vi "subplot_type.vi"(10 "数组":refnum<vi>[](array[refnum]), 11 "枚举":enum16{"1", "11", "1/1", "12", "1/2", "2/2"}(ring)) -> ()   [LabVIEW 2018, in "UI.lvlib"]
uses:
  UI.lvlib
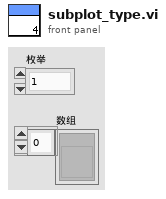
[diagram p1: front panel]
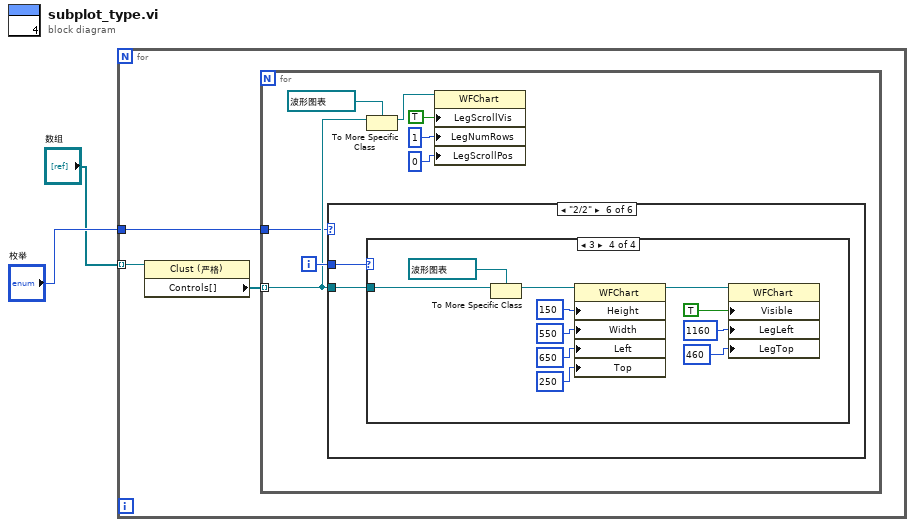
[diagram p0: block diagram]
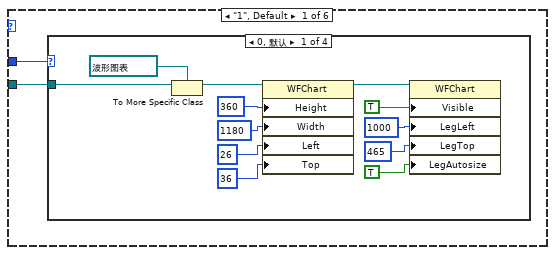
[diagram p2: hidden frame]
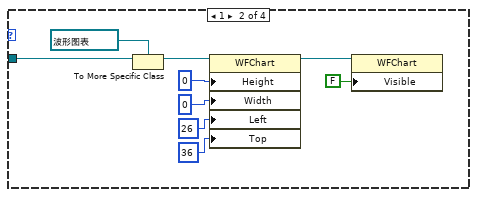
[diagram p3: hidden frame]
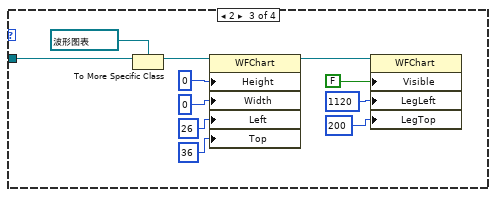
[diagram p4: hidden frame]
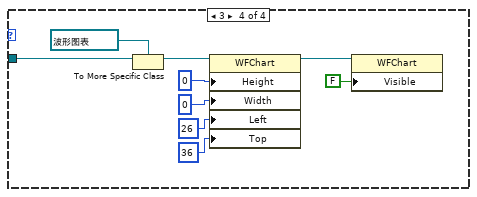
[diagram p5: hidden frame]
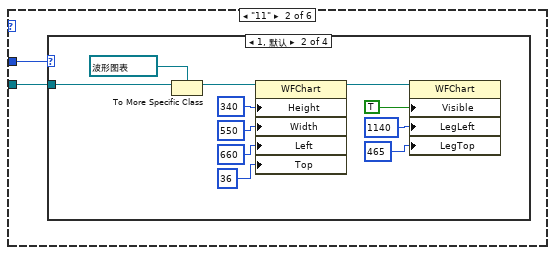
[diagram p6: hidden frame]
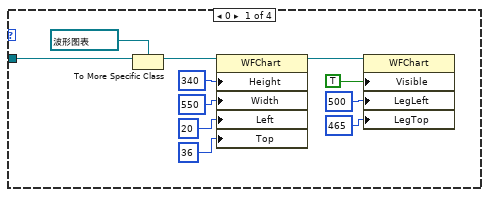
[diagram p7: hidden frame]
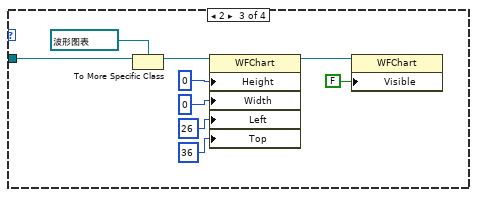
[diagram p8: hidden frame]
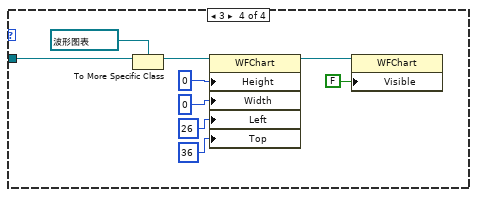
[diagram p9: hidden frame]
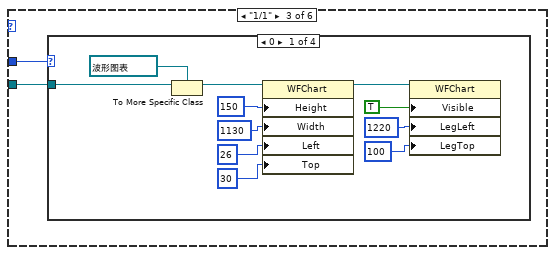
[diagram p10: hidden frame]
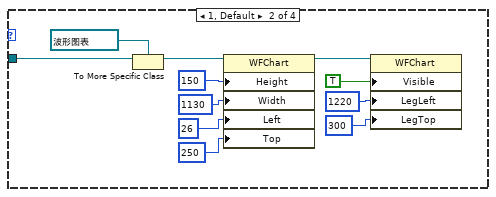
[diagram p11: hidden frame]
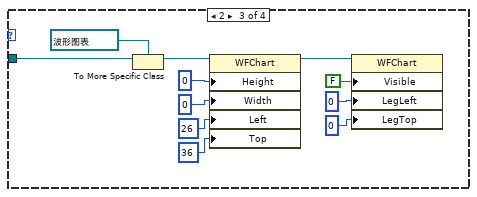
[diagram p12: hidden frame]
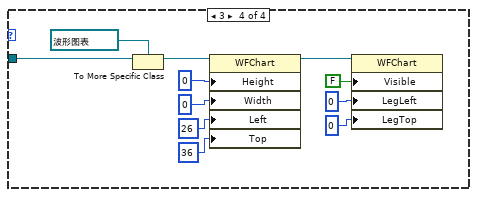
[diagram p13: hidden frame]
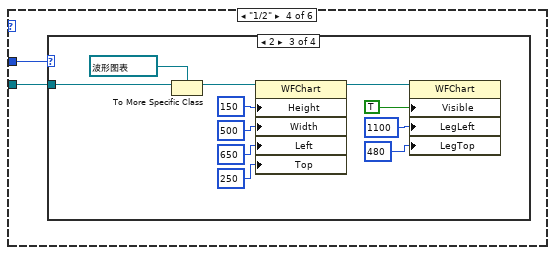
[diagram p14: hidden frame]
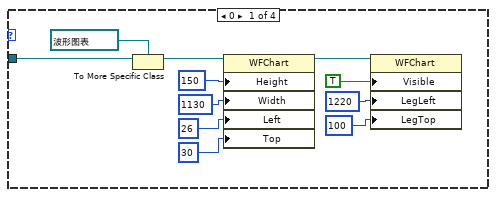
[diagram p15: hidden frame]
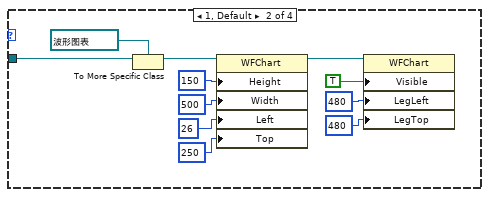
[diagram p16: hidden frame]
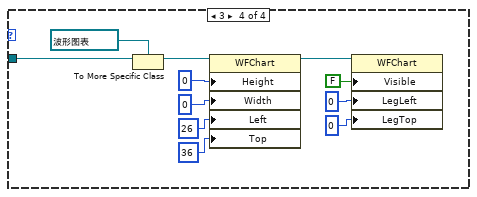
[diagram p17: hidden frame]
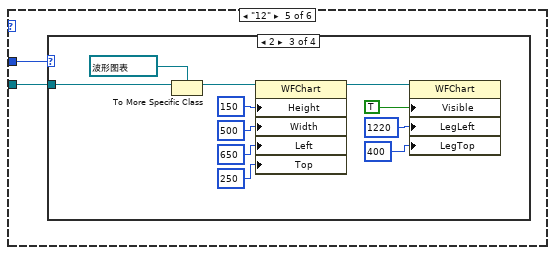
[diagram p18: hidden frame]
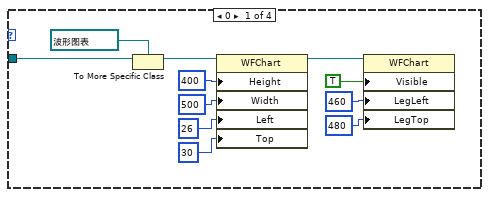
[diagram p19: hidden frame]
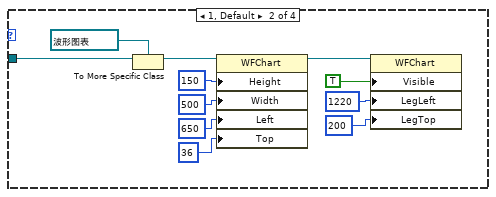
[diagram p20: hidden frame]
diagram:
  n1 = for {
    tunnel: "数组" -> [w4] mode=indexing
    tunnel: "枚举" -> [w3]
    n2 = property class="Clust (严格)"(reference=w4) -> ("Controls[]"=w5:refnum<vi>[])  [unwired: 1 in, 2 out]
    n3 = for {
      tunnel: w5 -> [w12] mode=indexing
      tunnel: w3 -> [w11]
      i -> [w13]
      n4 = case shown="\"2/2\"" w11 {
        tunnel: w13 -> [w15 w58 w100 w146 w192 w238]
        tunnel: w12 -> [w14 w57 w99 w145 w191 w237]
        frame "1", Default {
          n5 = case shown="0, 默认" w15 {
            tunnel: w14 -> [w23 w30 w43 w50]
            frame 0, Default {
              n6 = To More Specific Class(target class=refnum<vi> refnum ("特定类引用"), reference=w23) -> (specific class reference=w22:refnum<vi>)  [unwired: 1 in, 1 out]
              n7 = property class="WFChart"(reference=w22, "Height"=u32 360 ("绘图区域:大小:高度"), "Width"=u32 1180 ("绘图区域:大小:宽度"), "Left"=26 ("位置:居左"), "Top"=36 ("x")) -> (reference out=w17:refnum<vi>)  [unwired: 1 in, 1 out]
              n8 = property class="WFChart"(reference=w17, "Visible"=TRUE ("可见"), "LegLeft"=1000 ("图例:位置:居左"), "LegTop"=465 ("图例:位置:置顶"), "LegAutosize"=TRUE ("图例:自动调整大小")) -> ()  [unwired: 1 in, 2 out]
            }
            frame 1 {
              n9 = To More Specific Class(target class=refnum<vi> refnum ("特定类引用"), reference=w30) -> (specific class reference=w29:refnum<vi>)  [unwired: 1 in, 1 out]
              n10 = property class="WFChart"(reference=w29, "Height"=u32 0 ("绘图区域:大小:高度"), "Width"=u32 0 ("绘图区域:大小:宽度"), "Left"=26 ("位置:居左"), "Top"=36 ("x")) -> (reference out=w31:refnum<vi>)  [unwired: 1 in, 1 out]
              n11 = property class="WFChart"(reference=w31, "Visible"=FALSE ("可见")) -> ()  [unwired: 1 in, 2 out]
            }
            frame 2 {
              n12 = To More Specific Class(target class=refnum<vi> refnum ("特定类引用"), reference=w43) -> (specific class reference=w42:refnum<vi>)  [unwired: 1 in, 1 out]
              n13 = property class="WFChart"(reference=w42, "Height"=u32 0 ("绘图区域:大小:高度"), "Width"=u32 0 ("绘图区域:大小:宽度"), "Left"=26 ("位置:居左"), "Top"=36 ("x")) -> (reference out=w37:refnum<vi>)  [unwired: 1 in, 1 out]
              n14 = property class="WFChart"(reference=w37, "Visible"=FALSE ("可见"), "LegLeft"=1120 ("图例:位置:居左"), "LegTop"=200 ("图例:位置:置顶")) -> ()  [unwired: 1 in, 2 out]
            }
            frame 3 {
              n15 = To More Specific Class(target class=refnum<vi> refnum ("特定类引用"), reference=w50) -> (specific class reference=w49:refnum<vi>)  [unwired: 1 in, 1 out]
              n16 = property class="WFChart"(reference=w49, "Height"=u32 0 ("绘图区域:大小:高度"), "Width"=u32 0 ("绘图区域:大小:宽度"), "Left"=26 ("位置:居左"), "Top"=36 ("x")) -> (reference out=w51:refnum<vi>)  [unwired: 1 in, 1 out]
              n17 = property class="WFChart"(reference=w51, "Visible"=FALSE ("可见")) -> ()  [unwired: 1 in, 2 out]
            }
          }
        }
        frame "11" {
          n18 = case shown="1, 默认" w58 {
            tunnel: w57 -> [w65 w76 w83 w92]
            frame 0 {
              n19 = To More Specific Class(target class=refnum<vi> refnum ("特定类引用"), reference=w65) -> (specific class reference=w64:refnum<vi>)  [unwired: 1 in, 1 out]
              n20 = property class="WFChart"(reference=w64, "Height"=u32 340 ("绘图区域:大小:高度"), "Width"=u32 550 ("绘图区域:大小:宽度"), "Left"=20 ("位置:居左"), "Top"=36 ("x")) -> (reference out=w59:refnum<vi>)  [unwired: 1 in, 1 out]
              n21 = property class="WFChart"(reference=w59, "Visible"=TRUE ("可见"), "LegLeft"=500 ("图例:位置:居左"), "LegTop"=465 ("图例:位置:置顶")) -> ()  [unwired: 1 in, 2 out]
            }
            frame 1, Default {
              n22 = To More Specific Class(target class=refnum<vi> refnum ("特定类引用"), reference=w76) -> (specific class reference=w75:refnum<vi>)  [unwired: 1 in, 1 out]
              n23 = property class="WFChart"(reference=w75, "Height"=u32 340 ("绘图区域:大小:高度"), "Width"=u32 550 ("绘图区域:大小:宽度"), "Left"=660 ("位置:居左"), "Top"=36 ("x")) -> (reference out=w70:refnum<vi>)  [unwired: 1 in, 1 out]
              n24 = property class="WFChart"(reference=w70, "Visible"=TRUE ("可见"), "LegLeft"=1140 ("图例:位置:居左"), "LegTop"=465 ("图例:位置:置顶")) -> ()  [unwired: 1 in, 2 out]
            }
            frame 2 {
              n25 = To More Specific Class(target class=refnum<vi> refnum ("特定类引用"), reference=w83) -> (specific class reference=w82:refnum<vi>)  [unwired: 1 in, 1 out]
              n26 = property class="WFChart"(reference=w82, "Height"=u32 0 ("绘图区域:大小:高度"), "Width"=u32 0 ("绘图区域:大小:宽度"), "Left"=26 ("位置:居左"), "Top"=36 ("x")) -> (reference out=w84:refnum<vi>)  [unwired: 1 in, 1 out]
              n27 = property class="WFChart"(reference=w84, "Visible"=FALSE ("可见")) -> ()  [unwired: 1 in, 2 out]
            }
            frame 3 {
              n28 = To More Specific Class(target class=refnum<vi> refnum ("特定类引用"), reference=w92) -> (specific class reference=w91:refnum<vi>)  [unwired: 1 in, 1 out]
              n29 = property class="WFChart"(reference=w91, "Height"=u32 0 ("绘图区域:大小:高度"), "Width"=u32 0 ("绘图区域:大小:宽度"), "Left"=26 ("位置:居左"), "Top"=36 ("x")) -> (reference out=w93:refnum<vi>)  [unwired: 1 in, 1 out]
              n30 = property class="WFChart"(reference=w93, "Visible"=FALSE ("可见")) -> ()  [unwired: 1 in, 2 out]
            }
          }
        }
        frame "1/1" {
          n31 = case shown="0" w100 {
            tunnel: w99 -> [w107 w116 w129 w140]
            frame 0 {
              n32 = To More Specific Class(target class=refnum<vi> refnum ("特定类引用"), reference=w107) -> (specific class reference=w106:refnum<vi>)  [unwired: 1 in, 1 out]
              n33 = property class="WFChart"(reference=w106, "Height"=u32 150 ("绘图区域:大小:高度"), "Width"=u32 1130 ("绘图区域:大小:宽度"), "Left"=26 ("位置:居左"), "Top"=30 ("x")) -> (reference out=w101:refnum<vi>)  [unwired: 1 in, 1 out]
              n34 = property class="WFChart"(reference=w101, "Visible"=TRUE ("可见"), "LegLeft"=1220 ("图例:位置:居左"), "LegTop"=100 ("图例:位置:置顶")) -> ()  [unwired: 1 in, 2 out]
            }
            frame 1, Default {
              n35 = To More Specific Class(target class=refnum<vi> refnum ("特定类引用"), reference=w116) -> (specific class reference=w115:refnum<vi>)  [unwired: 1 in, 1 out]
              n36 = property class="WFChart"(reference=w115, "Height"=u32 150 ("绘图区域:大小:高度"), "Width"=u32 1130 ("绘图区域:大小:宽度"), "Left"=26 ("位置:居左"), "Top"=250 ("x")) -> (reference out=w117:refnum<vi>)  [unwired: 1 in, 1 out]
              n37 = property class="WFChart"(reference=w117, "Visible"=TRUE ("可见"), "LegLeft"=1220 ("图例:位置:居左"), "LegTop"=300 ("图例:位置:置顶")) -> ()  [unwired: 1 in, 2 out]
            }
            frame 2 {
              n38 = To More Specific Class(target class=refnum<vi> refnum ("特定类引用"), reference=w129) -> (specific class reference=w128:refnum<vi>)  [unwired: 1 in, 1 out]
              n39 = property class="WFChart"(reference=w128, "Height"=u32 0 ("绘图区域:大小:高度"), "Width"=u32 0 ("绘图区域:大小:宽度"), "Left"=26 ("位置:居左"), "Top"=36 ("x")) -> (reference out=w123:refnum<vi>)  [unwired: 1 in, 1 out]
              n40 = property class="WFChart"(reference=w123, "Visible"=FALSE ("可见"), "LegLeft"=0 ("图例:位置:居左"), "LegTop"=0 ("图例:位置:置顶")) -> ()  [unwired: 1 in, 2 out]
            }
            frame 3 {
              n41 = To More Specific Class(target class=refnum<vi> refnum ("特定类引用"), reference=w140) -> (specific class reference=w139:refnum<vi>)  [unwired: 1 in, 1 out]
              n42 = property class="WFChart"(reference=w139, "Height"=u32 0 ("绘图区域:大小:高度"), "Width"=u32 0 ("绘图区域:大小:宽度"), "Left"=26 ("位置:居左"), "Top"=36 ("x")) -> (reference out=w134:refnum<vi>)  [unwired: 1 in, 1 out]
              n43 = property class="WFChart"(reference=w134, "Visible"=FALSE ("可见"), "LegLeft"=0 ("图例:位置:居左"), "LegTop"=0 ("图例:位置:置顶")) -> ()  [unwired: 1 in, 2 out]
            }
          }
        }
        frame "1/2" {
          n44 = case shown="2" w146 {
            tunnel: w145 -> [w153 w162 w175 w186]
            frame 0 {
              n45 = To More Specific Class(target class=refnum<vi> refnum ("特定类引用"), reference=w153) -> (specific class reference=w152:refnum<vi>)  [unwired: 1 in, 1 out]
              n46 = property class="WFChart"(reference=w152, "Height"=u32 150 ("绘图区域:大小:高度"), "Width"=u32 1130 ("绘图区域:大小:宽度"), "Left"=26 ("位置:居左"), "Top"=30 ("x")) -> (reference out=w147:refnum<vi>)  [unwired: 1 in, 1 out]
              n47 = property class="WFChart"(reference=w147, "Visible"=TRUE ("可见"), "LegLeft"=1220 ("图例:位置:居左"), "LegTop"=100 ("图例:位置:置顶")) -> ()  [unwired: 1 in, 2 out]
            }
            frame 1, Default {
              n48 = To More Specific Class(target class=refnum<vi> refnum ("特定类引用"), reference=w162) -> (specific class reference=w161:refnum<vi>)  [unwired: 1 in, 1 out]
              n49 = property class="WFChart"(reference=w161, "Height"=u32 150 ("绘图区域:大小:高度"), "Width"=u32 500 ("绘图区域:大小:宽度"), "Left"=26 ("位置:居左"), "Top"=250 ("x")) -> (reference out=w163:refnum<vi>)  [unwired: 1 in, 1 out]
              n50 = property class="WFChart"(reference=w163, "Visible"=TRUE ("可见"), "LegLeft"=480 ("图例:位置:居左"), "LegTop"=480 ("图例:位置:置顶")) -> ()  [unwired: 1 in, 2 out]
            }
            frame 2 {
              n51 = To More Specific Class(target class=refnum<vi> refnum ("特定类引用"), reference=w175) -> (specific class reference=w174:refnum<vi>)  [unwired: 1 in, 1 out]
              n52 = property class="WFChart"(reference=w174, "Height"=u32 150 ("绘图区域:大小:高度"), "Width"=u32 500 ("绘图区域:大小:宽度"), "Left"=650 ("位置:居左"), "Top"=250 ("x")) -> (reference out=w169:refnum<vi>)  [unwired: 1 in, 1 out]
              n53 = property class="WFChart"(reference=w169, "Visible"=TRUE ("可见"), "LegLeft"=1100 ("图例:位置:居左"), "LegTop"=480 ("图例:位置:置顶")) -> ()  [unwired: 1 in, 2 out]
            }
            frame 3 {
              n54 = To More Specific Class(target class=refnum<vi> refnum ("特定类引用"), reference=w186) -> (specific class reference=w185:refnum<vi>)  [unwired: 1 in, 1 out]
              n55 = property class="WFChart"(reference=w185, "Height"=u32 0 ("绘图区域:大小:高度"), "Width"=u32 0 ("绘图区域:大小:宽度"), "Left"=26 ("位置:居左"), "Top"=36 ("x")) -> (reference out=w180:refnum<vi>)  [unwired: 1 in, 1 out]
              n56 = property class="WFChart"(reference=w180, "Visible"=FALSE ("可见"), "LegLeft"=0 ("图例:位置:居左"), "LegTop"=0 ("图例:位置:置顶")) -> ()  [unwired: 1 in, 2 out]
            }
          }
        }
        frame "12" {
          n57 = case shown="2" w192 {
            tunnel: w191 -> [w199 w208 w221 w232]
            frame 0 {
              n58 = To More Specific Class(target class=refnum<vi> refnum ("特定类引用"), reference=w199) -> (specific class reference=w198:refnum<vi>)  [unwired: 1 in, 1 out]
              n59 = property class="WFChart"(reference=w198, "Height"=u32 400 ("绘图区域:大小:高度"), "Width"=u32 500 ("绘图区域:大小:宽度"), "Left"=26 ("位置:居左"), "Top"=30 ("x")) -> (reference out=w193:refnum<vi>)  [unwired: 1 in, 1 out]
              n60 = property class="WFChart"(reference=w193, "Visible"=TRUE ("可见"), "LegLeft"=460 ("图例:位置:居左"), "LegTop"=480 ("图例:位置:置顶")) -> ()  [unwired: 1 in, 2 out]
            }
            frame 1, Default {
              n61 = To More Specific Class(target class=refnum<vi> refnum ("特定类引用"), reference=w208) -> (specific class reference=w207:refnum<vi>)  [unwired: 1 in, 1 out]
              n62 = property class="WFChart"(reference=w207, "Height"=u32 150 ("绘图区域:大小:高度"), "Width"=u32 500 ("绘图区域:大小:宽度"), "Left"=650 ("位置:居左"), "Top"=36 ("x")) -> (reference out=w209:refnum<vi>)  [unwired: 1 in, 1 out]
              n63 = property class="WFChart"(reference=w209, "Visible"=TRUE ("可见"), "LegLeft"=1220 ("图例:位置:居左"), "LegTop"=200 ("图例:位置:置顶")) -> ()  [unwired: 1 in, 2 out]
            }
            frame 2 {
              n64 = To More Specific Class(target class=refnum<vi> refnum ("特定类引用"), reference=w221) -> (specific class reference=w220:refnum<vi>)  [unwired: 1 in, 1 out]
              n65 = property class="WFChart"(reference=w220, "Height"=u32 150 ("绘图区域:大小:高度"), "Width"=u32 500 ("绘图区域:大小:宽度"), "Left"=650 ("位置:居左"), "Top"=250 ("x")) -> (reference out=w215:refnum<vi>)  [unwired: 1 in, 1 out]
              n66 = property class="WFChart"(reference=w215, "Visible"=TRUE ("可见"), "LegLeft"=1220 ("图例:位置:居左"), "LegTop"=400 ("图例:位置:置顶")) -> ()  [unwired: 1 in, 2 out]
            }
            frame 3 {
              n67 = To More Specific Class(target class=refnum<vi> refnum ("特定类引用"), reference=w232) -> (specific class reference=w231:refnum<vi>)  [unwired: 1 in, 1 out]
              n68 = property class="WFChart"(reference=w231, "Height"=u32 0 ("绘图区域:大小:高度"), "Width"=u32 0 ("绘图区域:大小:宽度"), "Left"=26 ("位置:居左"), "Top"=36 ("x")) -> (reference out=w226:refnum<vi>)  [unwired: 1 in, 1 out]
              n69 = property class="WFChart"(reference=w226, "Visible"=FALSE ("可见"), "LegLeft"=0 ("图例:位置:居左"), "LegTop"=0 ("图例:位置:置顶")) -> ()  [unwired: 1 in, 2 out]
            }
          }
        }
        frame "2/2" {
          n70 = case shown="3" w238 {
            tunnel: w237 -> [w245 w254 w268 w278]
            frame 0 {
              n71 = To More Specific Class(target class=refnum<vi> refnum ("特定类引用"), reference=w245) -> (specific class reference=w244:refnum<vi>)  [unwired: 1 in, 1 out]
              n72 = property class="WFChart"(reference=w244, "Height"=u32 150 ("绘图区域:大小:高度"), "Width"=u32 550 ("绘图区域:大小:宽度"), "Left"=26 ("位置:居左"), "Top"=30 ("x")) -> (reference out=w239:refnum<vi>)  [unwired: 1 in, 1 out]
              n73 = property class="WFChart"(reference=w239, "Visible"=TRUE ("可见"), "LegLeft"=500 ("图例:位置:居左"), "LegTop"=250 ("图例:位置:置顶")) -> ()  [unwired: 1 in, 2 out]
            }
            frame 1, Default {
              n74 = To More Specific Class(target class=refnum<vi> refnum ("特定类引用"), reference=w254) -> (specific class reference=w253:refnum<vi>)  [unwired: 1 in, 1 out]
              n75 = property class="WFChart"(reference=w253, "Height"=u32 150 ("绘图区域:大小:高度"), "Width"=u32 550 ("绘图区域:大小:宽度"), "Left"=650 ("位置:居左"), "Top"=30 ("x")) -> (reference out=w255:refnum<vi>)  [unwired: 1 in, 1 out]
              n76 = property class="WFChart"(reference=w255, "Visible"=TRUE ("可见"), "LegLeft"=1160 ("图例:位置:居左"), "LegTop"=250 ("图例:位置:置顶")) -> ()  [unwired: 1 in, 2 out]
            }
            frame 2 {
              n77 = To More Specific Class(target class=refnum<vi> refnum ("特定类引用"), reference=w268) -> (specific class reference=w267:refnum<vi>)  [unwired: 1 in, 1 out]
              n78 = property class="WFChart"(reference=w267, "Height"=u32 150 ("绘图区域:大小:高度"), "Width"=u32 550 ("绘图区域:大小:宽度"), "Left"=26 ("位置:居左"), "Top"=250 ("x")) -> (reference out=w262:refnum<vi>)  [unwired: 1 in, 1 out]
              n79 = property class="WFChart"(reference=w262, "Visible"=TRUE ("可见"), "LegLeft"=500 ("图例:位置:居左"), "LegTop"=460 ("图例:位置:置顶")) -> ()  [unwired: 1 in, 2 out]
            }
            frame 3 {
              n80 = To More Specific Class(target class=refnum<vi> refnum ("特定类引用"), reference=w278) -> (specific class reference=w277:refnum<vi>)  [unwired: 1 in, 1 out]
              n81 = property class="WFChart"(reference=w277, "Height"=u32 150 ("绘图区域:大小:高度"), "Width"=u32 550 ("绘图区域:大小:宽度"), "Left"=650 ("位置:居左"), "Top"=250 ("x")) -> (reference out=w272:refnum<vi>)  [unwired: 1 in, 1 out]
              n82 = property class="WFChart"(reference=w272, "Visible"=TRUE ("可见"), "LegLeft"=1160 ("图例:位置:居左"), "LegTop"=460 ("图例:位置:置顶")) -> ()  [unwired: 1 in, 2 out]
            }
          }
        }
      }
      n83 = To More Specific Class(target class=refnum<vi> refnum ("特定类引用"), reference=w12) -> (specific class reference=w10:refnum<vi>)  [unwired: 1 in, 1 out]
      n84 = property class="WFChart"(reference=w10, "LegScrollVis"=TRUE ("图例:滚动条可见"), "LegNumRows"=u32 1 ("图例:行数"), "LegScrollPos"=u32 0 ("图例:滚动条位置")) -> ()  [unwired: 1 in, 2 out]
    }
  }
